vi "rename channel test.vi"() -> ()   [LabVIEW 2013, in "CVT tests.lvlib"]
uses:
  CVT tests.lvlib
  <vilib>/NI/Tag Bus Module Framework/channel/channel classification.ctl
  configuration/CVT configuration.lvclass
  <vilib>/NI/Tag Bus Module Framework/root configuration/TBM configuration.lvclass/TBM configuration.ctl
  configuration/CVT configuration.lvclass/CVT configuration.ctl
  <vilib>/NI/Tag Bus/tag/tag descriptor.lvclass/tag descriptor.ctl
  <vilib>/NI/Tag Bus Module Framework/root configuration/Read instance name.vi
  configuration/Write channels.vi
  <vilib>/NI/Tag Bus Module Framework/channel/TBM channel.lvclass
  <vilib>/NI/Tag Bus Module Framework/root configuration/TBM configuration.lvclass
  <vilib>/NI/Tag Bus/tag/tag descriptor.lvclass
panel:
  out "rename success":bool
  out "no err":errorcluster
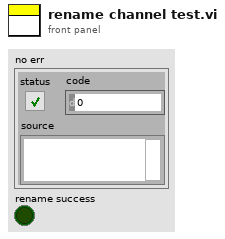
[diagram p1: front panel]
types:
  T1 = typedef "TBM channel.lvclass/channel classification.ctl" = enum16{"input data", "output data", "processing parameter", "processing result"}
  T2 = typedef "tag bus.lvlib/tag descriptor.lvclass/Data Type.ctl" = enum16{"Double", "Single", "I64", "I32", "I16", "I8", "U64", "U32", "U16", "U8", "Boolean", "String", "Array of Double", "Array of Single", "Array of I64", "Array of I32", "Array of I16", "Array of I8", "Array of U64", "Array of U32", "Array of U16", "Array of U8", "Array of Boolean", "Array of String"}
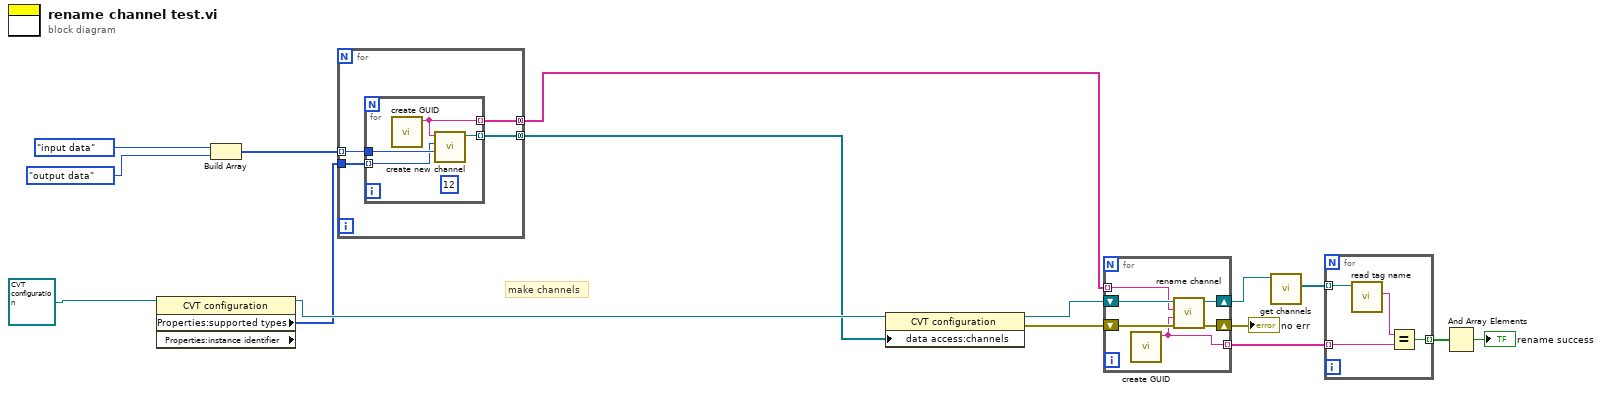
[diagram p0: block diagram]
diagram:
  # "make channels"
  n1 = property class="CVT configuration" props=["Properties:supported types", "Properties:instance identifier"](reference=refnum<class "CVT configuration.lvclass"> refnum ("tag bus configurable plugin module configuration")) -> (reference out=w13:refnum<class "CVT configuration.lvclass">, "Properties:supported types"=w12:T2[])  [unwired: 1 in, 2 out]
  n2 = Build Array(channel_classification."input data" ("channel classification"), channel_classification."output data" ("channel classification")) -> (w14:T1[])
  n3 = for {
    tunnel: w14 -> [w20] mode=indexing
    tunnel: [w18] -> w1 mode=concatenating
    tunnel: w12 -> [w19]
    tunnel: [w17] -> w11 mode=concatenating
    n4 = for {
      tunnel: w20 -> [w23]
      tunnel: [w24] -> w18 mode=indexing
      tunnel: w19 -> [w22] mode=indexing
      tunnel: [w21] -> w17 mode=indexing
      (unwired) 12
      n5 = call <vilib>:"create GUID.vi"() -> ("uuid"=w21:string)  [unwired: 11 in]
      n6 = call <vilib>:"create new channel.vi"("channel classification"=w23, "data type"=w22, "channel name"=w21) -> ("channel"=w24:refnum<class "TBM channel.lvclass">)  [unwired: 8 in]
    }
  }
  n7 = property class="CVT configuration"(reference=w13, "data access:channels"=w1) -> (reference out=w2:refnum<class "CVT configuration.lvclass">, error out=w3:errorcluster)  [unwired: 1 in]
  n8 = for {
    tunnel: w11 -> [w26] mode=indexing
    shift-right: [w27] -> w10
    shift-left: w2 -> [w30]
    shift-right: [w28] -> w8
    shift-left: w3 -> [w29]
    tunnel: [w25] -> w9 mode=indexing
    n9 = call <vilib>:"create GUID.vi"() -> ("uuid"=w25:string)  [unwired: 11 in]
    n10 = call "rename channel.vi"("error in"=w29, "new name"=w25, "old name"=w26, "CVT configuration in"=w30) -> ("error out"=w28:errorcluster, "CVT configuration out"=w27:refnum<class "CVT configuration.lvclass">)  [unwired: 6 in]
  }
  "no err" <- w8
  n11 = call-dynamic "get channels.vi"("CVT configuration in"=w10) -> ("channels"=w7:refnum<class "TBM channel.lvclass">[])  [unwired: 9 in, 1 out]
  n12 = for {
    tunnel: w9 -> [w33] mode=indexing
    tunnel: w7 -> [w34] mode=indexing
    tunnel: [w31] -> w6 mode=indexing
    n13 = call <vilib>:"read tag name.vi"("system tag in"=w34) -> ("name"=w32:string)  [unwired: 8 in, 2 out]
    n14 = Equal?(x=w32, y=w33) -> (x = y?=w31:bool)
  }
  n15 = And Array Elements(Boolean array=w6) -> (logical AND=→"rename success":bool)
